vi "Match Tips.vi"(8 "error in (no error)":errorcluster, 10 "Tip Matching Options":T1, 11 "Tips":T3[](array[typedef]) {"ROI Descriptor"."Contours"."Type" items=["No Selection", "Point", "Line", "Rectangle", "Oval", "Polygon", "Freehand Region", "Annulus", "Unused2", "Unused3", "Broken Line", "Freehand Line", "Rotated Rectangle"]; "Point"."Y" format="%.2f"; "Point"."X" format="%.2f"}) -> (0 "error out":errorcluster, 3 "Tracks":T2[](array[typedef]) {"ROI Descriptor"."Contours"."Type" items=["No Selection", "Point", "Line", "Rectangle", "Oval", "Polygon", "Freehand Region", "Annulus", "Unused2", "Unused3", "Broken Line", "Freehand Line", "Rotated Rectangle"]; "Tip 2"."ROI Descriptor"."Contours"."Type" items=["No Selection", "Point", "Line", "Rectangle", "Oval", "Polygon", "Freehand Region", "Annulus", "Unused2", "Unused3", "Broken Line", "Freehand Line", "Rotated Rectangle"]; "Tip 2"."Point"."Y" format="%.2f"; "Tip 2"."Point"."X" format="%.2f"; "Tip 1"."ROI Descriptor"."Contours"."Type" items=["No Selection", "Point", "Line", "Rectangle", "Oval", "Polygon", "Freehand Region", "Annulus", "Unused2", "Unused3", "Broken Line", "Freehand Line", "Rotated Rectangle"]; "Tip 1"."Point"."Y" format="%.2f"; "Tip 1"."Point"."X" format="%.2f"})   [LabVIEW 2013]
uses:
  Controls/Tip.ctl
  Controls/Track.ctl
  C:/Users/Andrew/Documents/Apatite to Zircon Code/Track Finding/Tip and Track Finding/TrackFinding.dll
  TrackFinding.dll
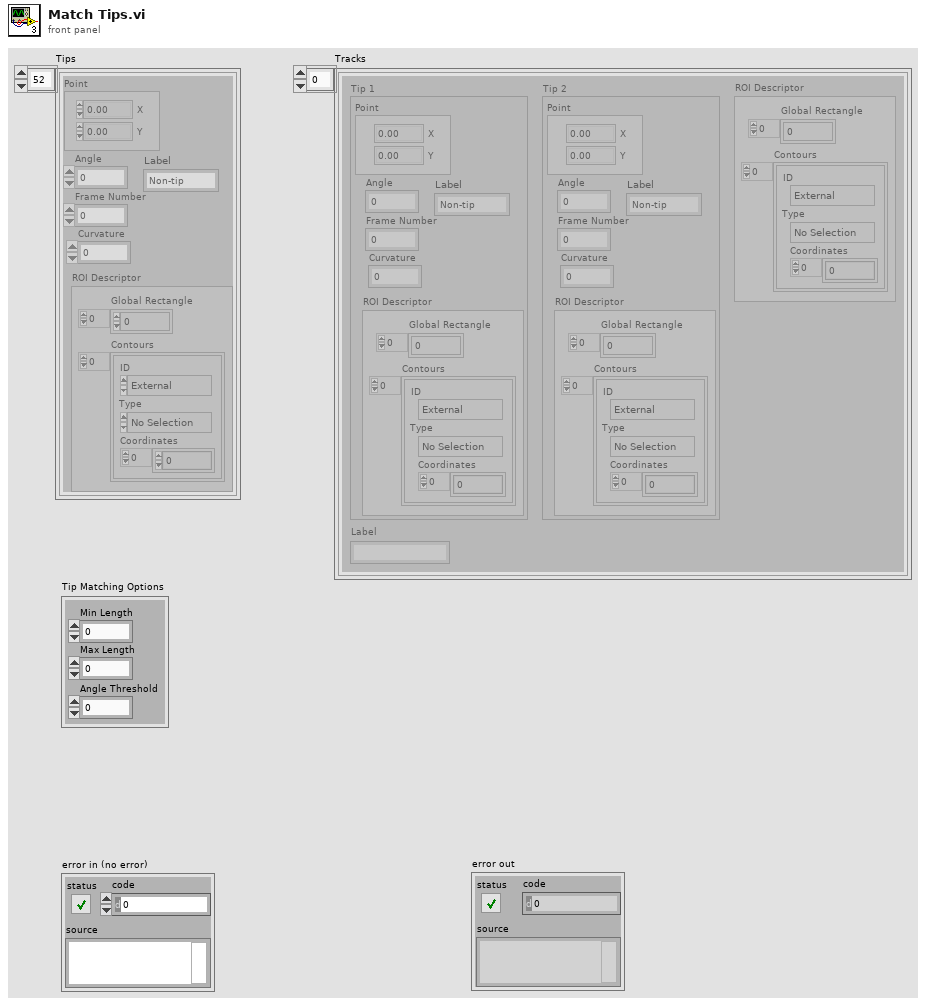
[diagram p1: front panel]
types:
  T1 = cluster{"Min Length":dbl, "Max Length":dbl, "Angle Threshold":dbl}
  T2 = typedef "Track.ctl" = cluster{"Tip 1":T3, "Tip 2":T3, "Label":string, "ROI Descriptor":T5}
  T3 = typedef "Tip.ctl" = cluster{"Point":T4, "Angle":dbl, "Frame Number":i32, "ROI Descriptor":T5, "Curvature":dbl, "Label":string}
  T4 = typedef "IMAQ Point" = cluster{"X":sgl, "Y":sgl}
  T5 = typedef "ROI Descriptor" = cluster{"Global Rectangle":i32[], "Contours":cluster{"ID":enum32{"External", "Internal"}, "Type":u32, "Coordinates":i32[]}[]}
  T6 = typedef "IMAQ Rectangle" = cluster{"Left":i32, "Top":i32, "Right":i32, "Bottom":i32, "Rotation":dbl}
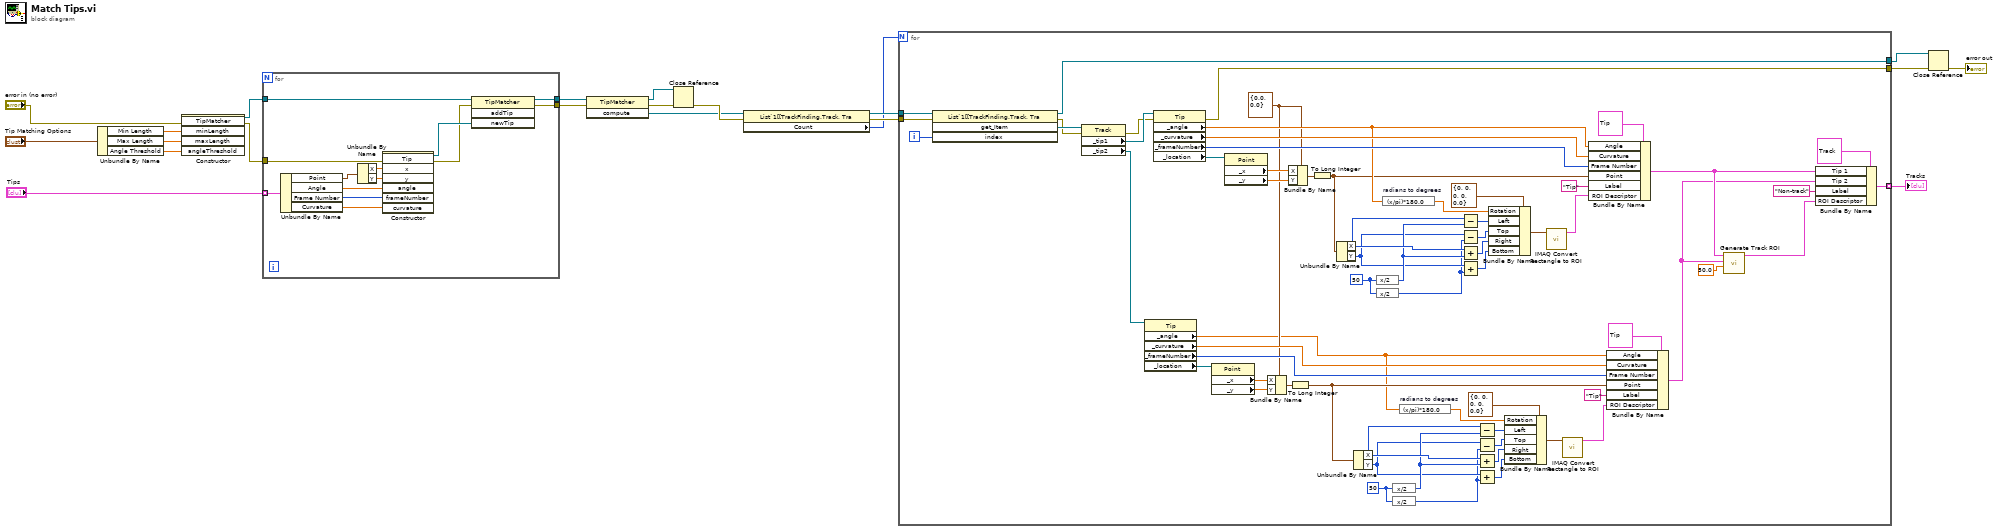
[diagram p0: block diagram]
diagram:
  n1 = Unbundle By Name("Tip Matching Options") -> ("Min Length"=w6:dbl, "Max Length"=w5:dbl, "Angle Threshold"=w4:dbl)
  n2 = constructor class="TipMatcher"(error in="error in (no error)", "minLength"=w6, "maxLength"=w5, "angleThreshold"=w4) -> (reference out=w2:refnum<k24>, error out=w1:errorcluster)  [unwired: 2 in, 4 out]
  n3 = for {
    tunnel: "Tips" -> [w34] mode=indexing
    tunnel: [w25] -> w19
    tunnel: [w24] -> w18
    tunnel: w2 -> [w23]
    tunnel: w1 -> [w22]
    n4 = Unbundle By Name(w34) -> ("Point"=w33:T4, "Angle"=w30:dbl, "Frame Number"=w29:i32, "Curvature"=w28:dbl)
    n5 = Unbundle By Name(w33) -> ("X"=w32:sgl, "Y"=w31:sgl)
    n6 = constructor class="Tip"(error in=w22, "x"=w32, "y"=w31, "angle"=w30, "frameNumber"=w29, "curvature"=w28) -> (reference out=w27:refnum<k24>, error out=w26:errorcluster)  [unwired: 2 in, 6 out]
    n7 = invoke class="TipMatcher" method="addTip"(reference=w23, error in=w26, "newTip"=w27) -> (reference out=w25:refnum<k24>, error out=w24:errorcluster)  [unwired: 1 in, 2 out]
  }
  n8 = invoke class="TipMatcher" method="compute"(reference=w19, error in=w18) -> (reference out=w16:refnum<k24>, error out=w17:errorcluster, "compute"=w14:refnum<k24>)  [unwired: 1 in]
  n9 = Close Reference(reference=w16, error in (no error)=w17) -> (error out=w15:errorcluster)
  n10 = property class="List`1[[TrackFinding.Track, Tra"(reference=w14, error in=w15) -> (reference out=w12:refnum<k24>, error out=w13:errorcluster, "Count"=w11:i32)
  n11 = for {
    N: w11 -> [_]
    tunnel: w12 -> [w98]
    tunnel: w13 -> [w95]
    tunnel: [w83] -> w9
    tunnel: [w78] -> w10
    tunnel: [w77] -> w8 mode=indexing
    i -> [w97]
    w45 = 50
    w59 = 50
    w57 = T4 {"X"=0.0, "Y"=0.0} ("Point")
    n12 = invoke class="List`1[[TrackFinding.Track, Tra" method="get_Item"(reference=w98, error in=w95, "index"=w97) -> (reference out=w83:refnum<k24>, error out=w94:errorcluster, "get_Item"=w96:refnum<k24>)  [unwired: 1 in, 1 out]
    n13 = property class="Track"(reference=w96, error in=w94) -> (error out=w84:errorcluster, "_tip1"=w93:refnum<k24>, "_tip2"=w91:refnum<k24>)  [unwired: 1 out]
    n14 = property class="Tip"(reference=w91) -> ("_angle"=w41:dbl, "_curvature"=w81:dbl, "_frameNumber"=w82:i32, "_location"=w90:refnum<k24>)  [unwired: 1 in, 2 out]
    n15 = property class="Tip"(reference=w93, error in=w84) -> (error out=w78:errorcluster, "_angle"=w61:dbl, "_curvature"=w80:dbl, "_frameNumber"=w79:i32, "_location"=w92:refnum<k24>)  [unwired: 1 out]
    n16 = property class="Point"(reference=w90) -> ("_x"=w86:dbl, "_y"=w85:dbl)  [unwired: 1 in, 2 out]
    n17 = property class="Point"(reference=w92) -> ("_x"=w88:dbl, "_y"=w87:dbl)  [unwired: 1 in, 2 out]
    n18 = Bundle By Name(cluster=w57, "X"=w86, "Y"=w85) -> (w58:T4)
    n19 = Bundle By Name(cluster=w57, "X"=w88, "Y"=w87) -> (w89:T4)
    n20 = To Long Integer(number=w58) -> (32bit integer=w42:cluster{"X":i32, "Y":i32})
    n21 = To Long Integer(number=w89) -> (32bit integer=w60:cluster{"X":i32, "Y":i32})
    n22 = Unbundle By Name(w60) -> ("X"=w73:i32, "Y"=w71:i32)
    n23 = Unbundle By Name(w42) -> ("X"=w56:i32, "Y"=w54:i32)
    n24 = expression code="x/2"(w59) -> (w72:i32)
    n25 = expression code="x/2"(w59) -> (w70:i32)
    n26 = expression code="(x/pi)*180.0" "radians to degrees"(w61) -> (w64:dbl)
    n27 = expression code="x/2"(w45) -> (w55:i32)
    n28 = expression code="x/2"(w45) -> (w53:i32)
    n29 = expression code="(x/pi)*180.0" "radians to degrees"(w41) -> (w47:dbl)
    n30 = Subtract(x=w73, y=w72) -> (x-y=w67:i32)
    n31 = Subtract(x=w71, y=w70) -> (x-y=w68:i32)
    n32 = Add(x=w73, y=w72) -> (x+y=w65:i32)
    n33 = Add(x=w71, y=w70) -> (x+y=w66:i32)
    n34 = Subtract(x=w56, y=w55) -> (x-y=w50:i32)
    n35 = Subtract(x=w54, y=w53) -> (x-y=w51:i32)
    n36 = Add(x=w56, y=w55) -> (x+y=w48:i32)
    n37 = Add(x=w54, y=w53) -> (x+y=w49:i32)
    n38 = Bundle By Name(cluster=T6 {"Left"=0, "Top"=0, "Right"=0, "Bottom"=0, "Rotation"=0.0} ("Rectangle"), "Rotation"=w64, "Left"=w67, "Top"=w68, "Right"=w65, "Bottom"=w66) -> (w63:T6)
    n39 = Bundle By Name(cluster=T6 {"Left"=0, "Top"=0, "Right"=0, "Bottom"=0, "Rotation"=0.0} ("Rectangle"), "Rotation"=w47, "Left"=w50, "Top"=w51, "Right"=w48, "Bottom"=w49) -> (w46:T6)
    n40 = call "IMAQ Convert Rectangle to ROI"("Rectangle"=w63) -> ("ROI Descriptor"=w62:T5)  [unwired: 8 in, 1 out]
    n41 = call "IMAQ Convert Rectangle to ROI"("Rectangle"=w46) -> ("ROI Descriptor"=w43:T5)  [unwired: 8 in, 1 out]
    n42 = Bundle By Name(cluster=T3 {"Point"={"X"=0.0, "Y"=0.0}, "Angle"=0.0, "Frame Number"=0, "ROI Descriptor"={"Global Rectangle"=[], "Contours"=[]}, "Curvature"=0.0, "Label"="Non-tip"} ("Tip"), "Angle"=w61, "Curvature"=w80, "Frame Number"=w79, "Point"=w60, "Label"="Tip", "ROI Descriptor"=w62) -> (w37:T3)
    n43 = Bundle By Name(cluster=T3 {"Point"={"X"=0.0, "Y"=0.0}, "Angle"=0.0, "Frame Number"=0, "ROI Descriptor"={"Global Rectangle"=[], "Contours"=[]}, "Curvature"=0.0, "Label"="Non-tip"} ("Tip"), "Angle"=w41, "Curvature"=w81, "Frame Number"=w82, "Point"=w42, "Label"="Tip", "ROI Descriptor"=w43) -> (w36:T3)
    n44 = call "Generate Track ROI.vi"("ROI Width"=50.0, "Tip 2"=w36, "Tip 1"=w37) -> ("Track ROI"=w38:T5)  [unwired: 7 in, 1 out]
    n45 = Bundle By Name(cluster=T2 {"Tip 1"={"Point"={"X"=0.0, "Y"=0.0}, "Angle"=0.0, "Frame Number"=0, "ROI Descriptor"={"Global Rectangle"=[], "Contours"=[]}, "Curvature"=0.0, "Label"="Non-tip"}, "Tip 2"={"Point"={"X"=0.0, "Y"=0.0}, "Angle"=0.0, "Frame Number"=0, "ROI Descriptor"={"Global Rectangle"=[], "Contours"=[]}, "Curvature"=0.0, "Label"="Non-tip"}, "Label"="", "ROI Descriptor"={"Global Rectangle"=[], "Contours"=[]}} ("Track"), "Tip 1"=w37, "Tip 2"=w36, "Label"="Non-track", "ROI Descriptor"=w38) -> (w77:T2)
  }
  "Tracks" <- w8
  n46 = Close Reference(reference=w9, error in (no error)=w10) -> (error out=→"error out":errorcluster)
